vi "PopulateTreeSumaryWithGlyphManager.vi"(8 "error in":errorcluster, 9 "glyph manager":T1, 10 "summary":T3[](array[typedef]), 11 "tree ref in":refnum<vi>) -> (0 "error out":errorcluster, 1 "glyph manager out":T1)   [LabVIEW 2013, in "NISE_CEF_TreeControl.lvlib"]
doc: "This VI will populate the tree control with the summary from the nodes. Use this when adding new nodes to tree"
uses:
  NISE_CEF_TreeControl.lvlib
  Node/Summary.ctl
  glyph manager/glyph manager.ctl
  <vilib>/picture/picture.llb/imagedata.ctl
  glyph manager/glyph manager.lvlib
  Node/NISE_CEF_Node.lvclass
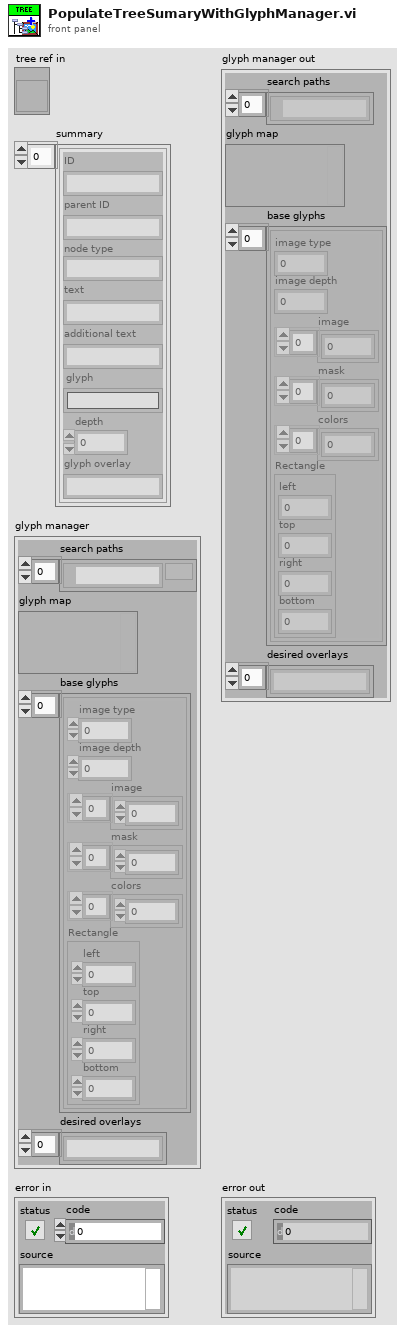
[diagram p1: front panel]
types:
  T1 = typedef "glyph manager.lvlib/glyph manager.ctl" = cluster{"search paths":path[], "glyph map":variant, "base glyphs":T2[], "desired overlays":string[]}
  T2 = typedef "imagedata.ctl" = cluster{"image type":i32, "image depth":i32, "image":u8[], "mask":u8[], "colors":u32[], "Rectangle":cluster{"left":i16, "top":i16, "right":i16, "bottom":i16}}
  T3 = typedef "NISE_CEF_Node.lvclass/Summary.ctl" = cluster{"ID":string, "parent ID":string, "node type":string, "text":string, "additional text":string, "glyph":string, "depth":i32, "glyph overlay":string}
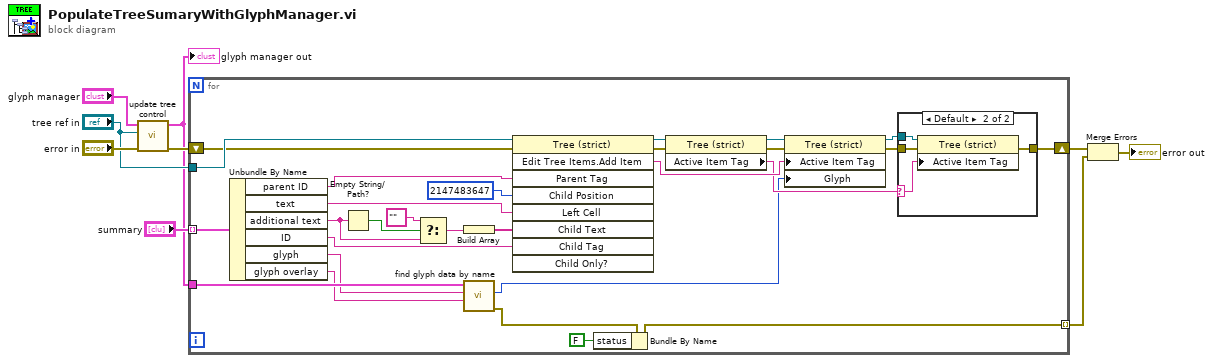
[diagram p0: block diagram]
diagram:
  n1 = call "update tree control.vi"("error in"="error in", "tree reference"="tree ref in", "glyph manager in"="glyph manager") -> ("error out"=w5:errorcluster, "glyph manager out"=w1:T1)  [unwired: 7 in]
  "glyph manager out" <- w1
  n2 = for {
    tunnel: "summary" -> [w22] mode=indexing
    shift-right: [w19] -> w2
    shift-left: w5 -> [w20]
    tunnel: [w11] -> w7 mode=indexing
    tunnel: "tree ref in" -> [w21]
    tunnel: w1 -> [w16]
    n3 = Unbundle By Name(w22) -> ("parent ID"=w37:string, "text"=w23:string, "additional text"=w18:string, "ID"=w34:string, "glyph"=w15:string, "glyph overlay"=w14:string)
    n4 = Empty String/Path?(string/path=w18) -> (empty?=w17:bool)
    n5 = Select(t="", s=w17, f=w18) -> (s? t:f=w32:string)
    n6 = Build Array(w32) -> (w35:string[])
    n7 = call "find glyph data by name.vi"("overlay"=w14, "name"=w15, "glyph manager in"=w16) -> ("error out"=w13:errorcluster, "symbol index"=w12:i32)  [unwired: 5 in, 2 out]
    n8 = invoke class="Tree (strict)" method="Edit Tree Items.Add Item"(reference=w21, error in=w20, "Parent Tag"=w37, "Child Position"=2147483647 ("child Position"), "Left Cell"=w23, "Child Text"=w35, "Child Tag"=w34) -> (reference out=w31:refnum<vi>, error out=w30:errorcluster, "Edit Tree Items:Add Item"=w27:string)  [unwired: 2 in, 6 out]
    n9 = Bundle By Name(cluster=w13, "status"=FALSE) -> (w11:errorcluster)
    n10 = property class="Tree (strict)"(reference=w31, error in=w30) -> (reference out=w29:refnum<vi>, error out=w28:errorcluster, "Active Item Tag"=w24:string)
    n11 = property class="Tree (strict)"(reference=w29, error in=w28, "Active Item Tag"=w27, "Glyph"=w12) -> (reference out=w26:refnum<vi>, error out=w25:errorcluster)
    n12 = case shown="Default" w24 {
      selector: w24 -> [_ w40]
      tunnel: w26 -> [_ w42]
      tunnel: w25 -> [w38 w41]
      tunnel: [w38 w39] -> w19
      frame "" {
      }
      frame Default {
        n13 = property class="Tree (strict)"(reference=w42, error in=w41, "Active Item Tag"=w40) -> (error out=w39:errorcluster)  [unwired: 1 out]
      }
    }
  }
  n14 = Merge Errors(w2, w7) -> (→"error out":errorcluster)
